vi "数据查询_仪器数据.vi"() -> ()   [LabVIEW 2016, in "数据查询.lvlib"]
uses:
  <vilib>/Utility/miscctls.llb/LVPointTypeDef.ctl
  <vilib>/Utility/miscctls.llb/LVRowAndColumnUnsignedTypeDef.ctl
  <userlib>/_OpenG.lib/array/array.llb/Sort 2D Array (String)__ogtk.vi
panel:
  in  "是否剔除异常数据":bool
  in  "数据类型":string(combo)="全部数据"
  in  "列表框":i32(listbox)
  out "布尔":bool
  in  "页":i32 format="第%.0f页"
  in  "每页条数":i32=1000
  in  "向后按钮":bool
  in  "向前按钮":bool
  in  "导出":bool
  in  "测量模式":string(combo)="全部数据"
  in  "查询":bool
  in  "结束日期":string="2050/01/01"
  in  "起始日期":string="2010/01/01"
  out "数据表":string[][](table)
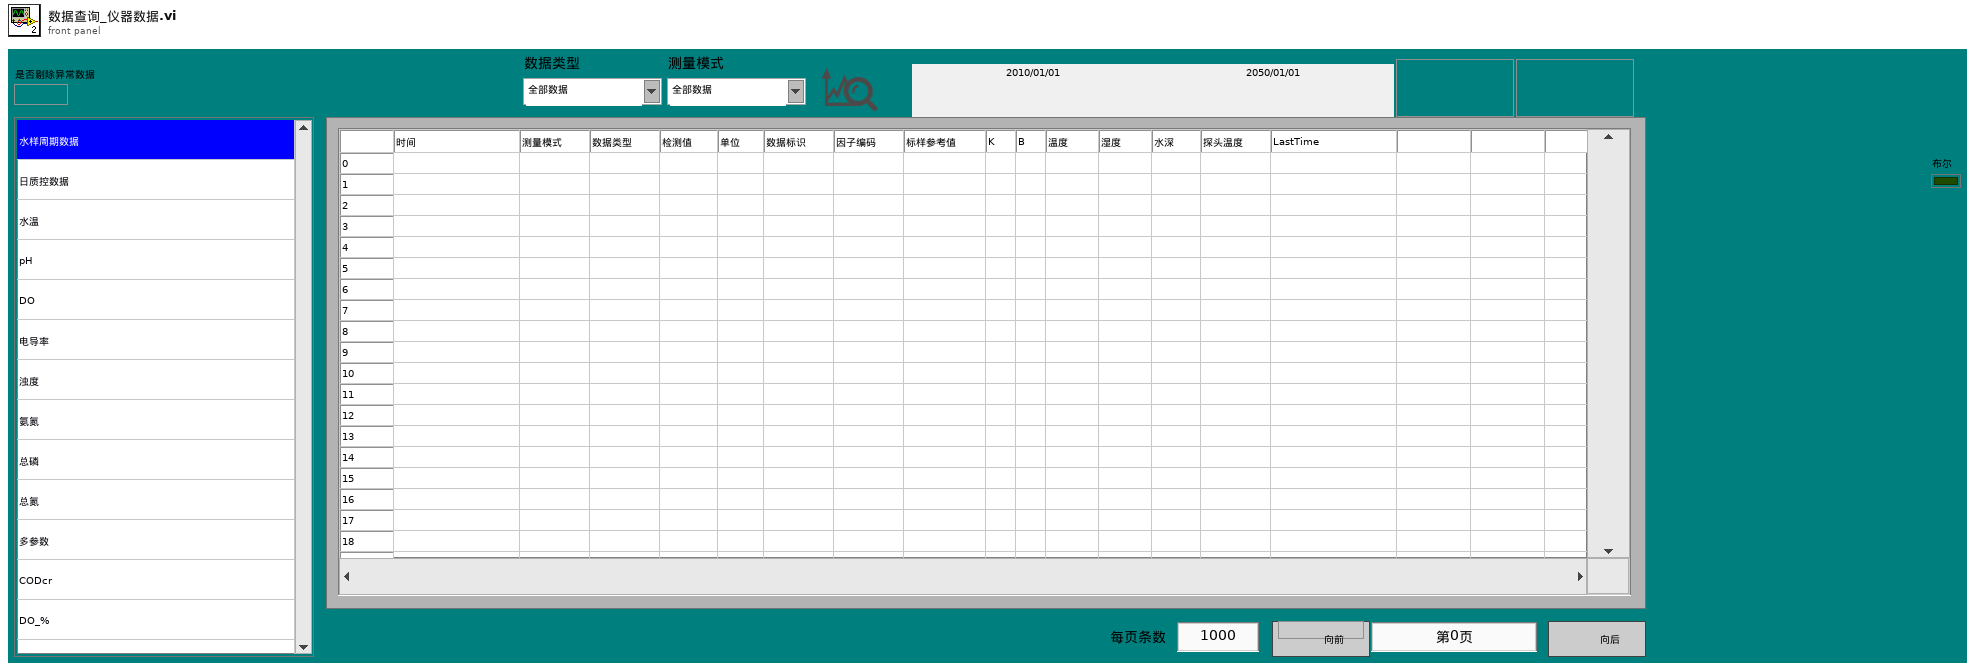
[diagram p1: front panel]
types:
  T1 = typedef "LVPointTypeDef.ctl" = cluster{"Horizontal":i16, "Vertical":i16}
  T2 = typedef "LVDateTimeRec.ctl" = cluster{"秒数的小数部分":dbl, "秒":i32, "分":i32, "时":i32, "日":i32, "月":i32, "年":i32, "天数（周）":i32, "天数（年）":i32, "DST":i32}
  T3 = enum8{"Enabled", "Disabled", "Disabled and Grayed Out"}
  T4 = typedef "LVRowAndColumnUnsignedTypeDef.ctl" = cluster{"Row":u32, "Column":u32}
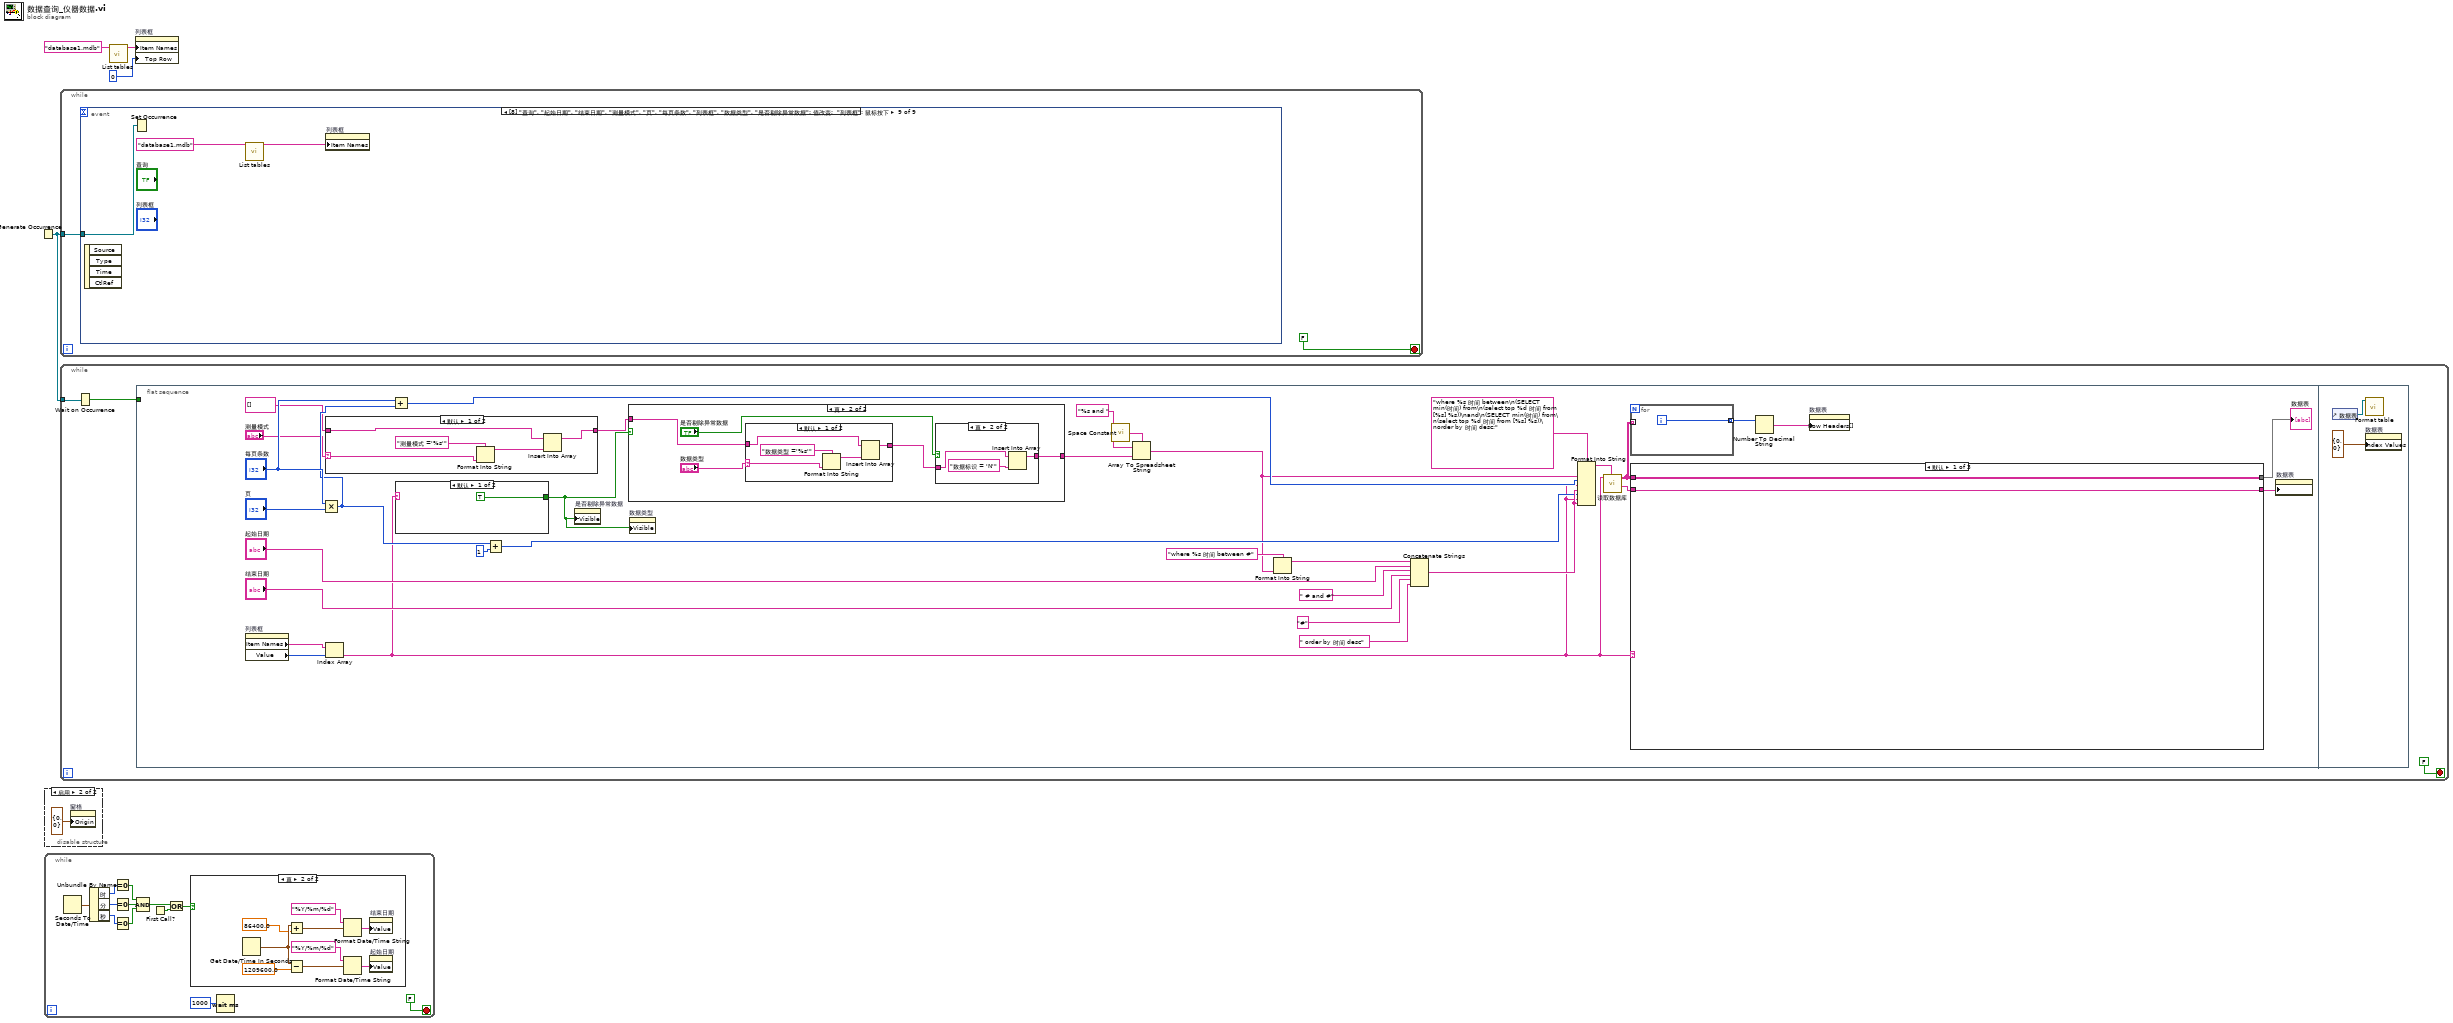
[diagram p0: block diagram]
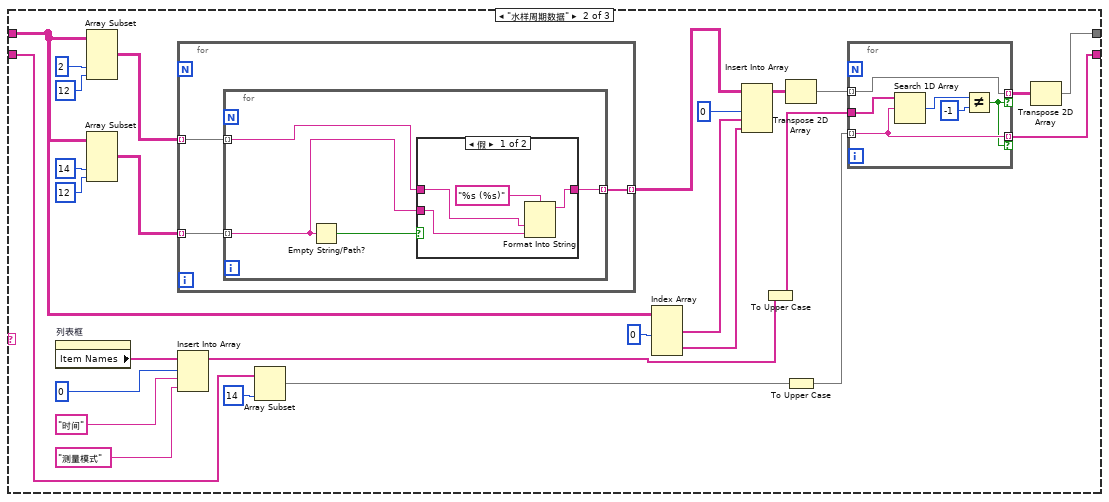
[diagram p7: hidden frame]
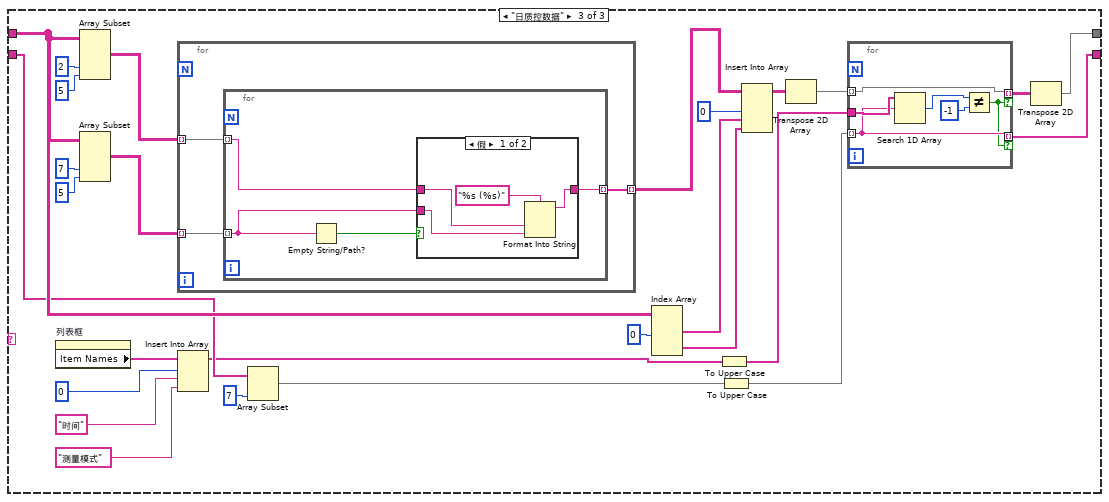
[diagram p9: hidden frame]
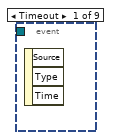
[diagram p12: hidden frame]
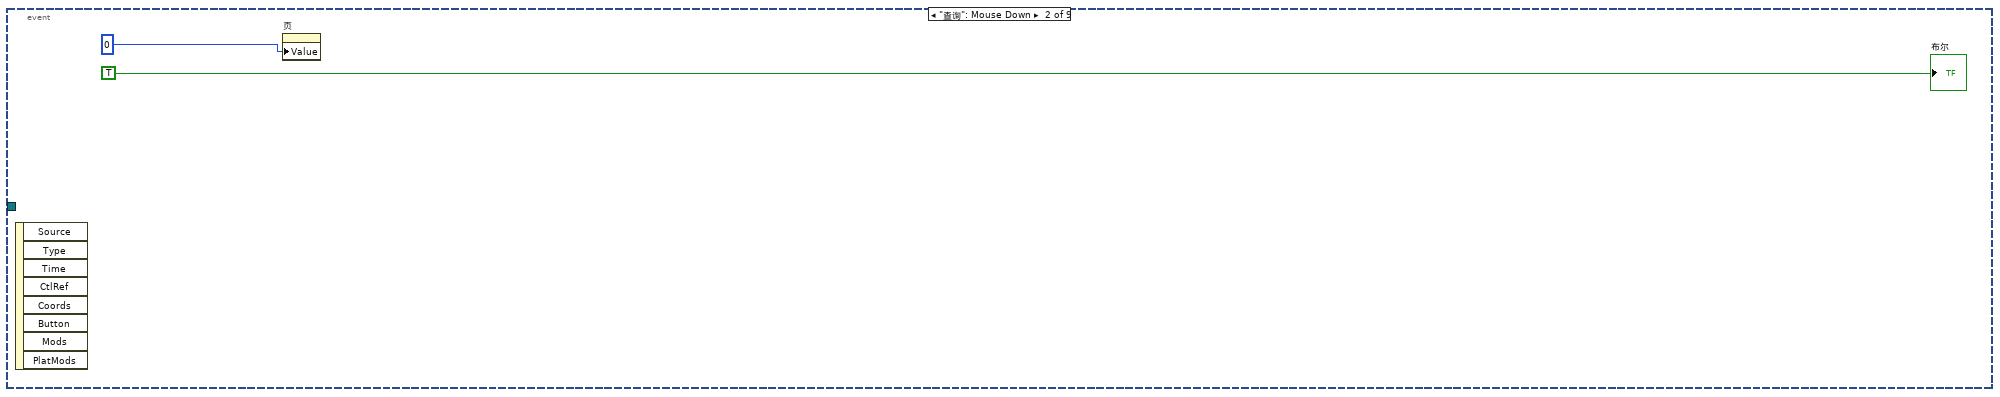
[diagram p13: hidden frame]
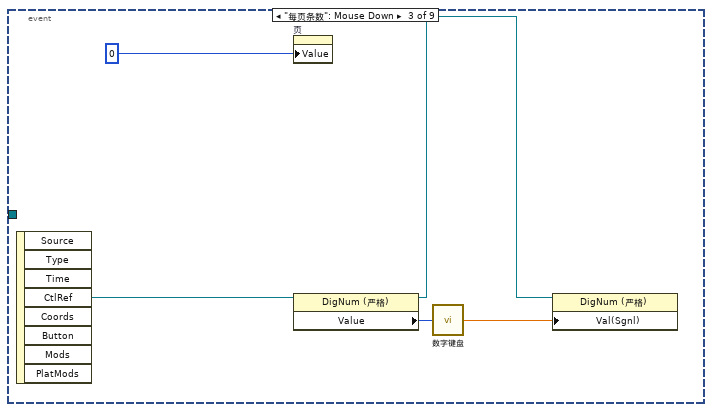
[diagram p14: hidden frame]
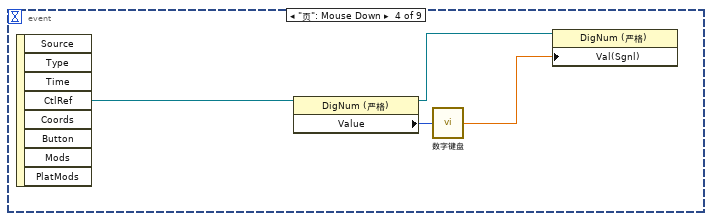
[diagram p15: hidden frame]
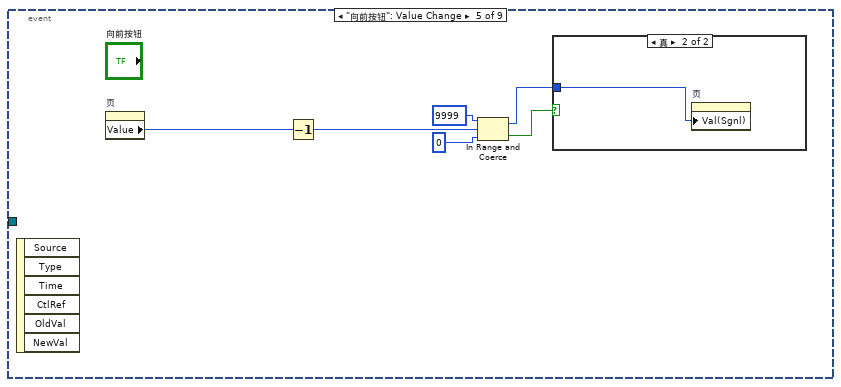
[diagram p16: hidden frame]
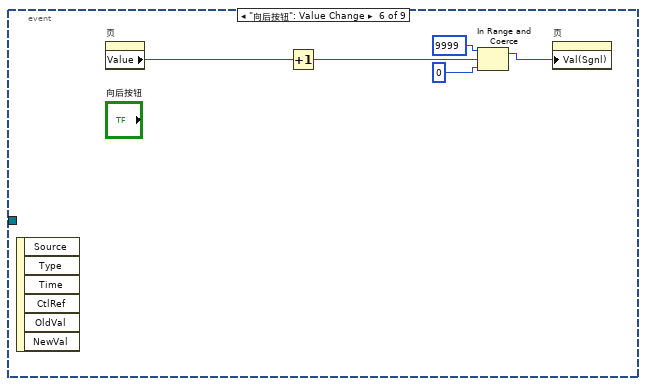
[diagram p18: hidden frame]
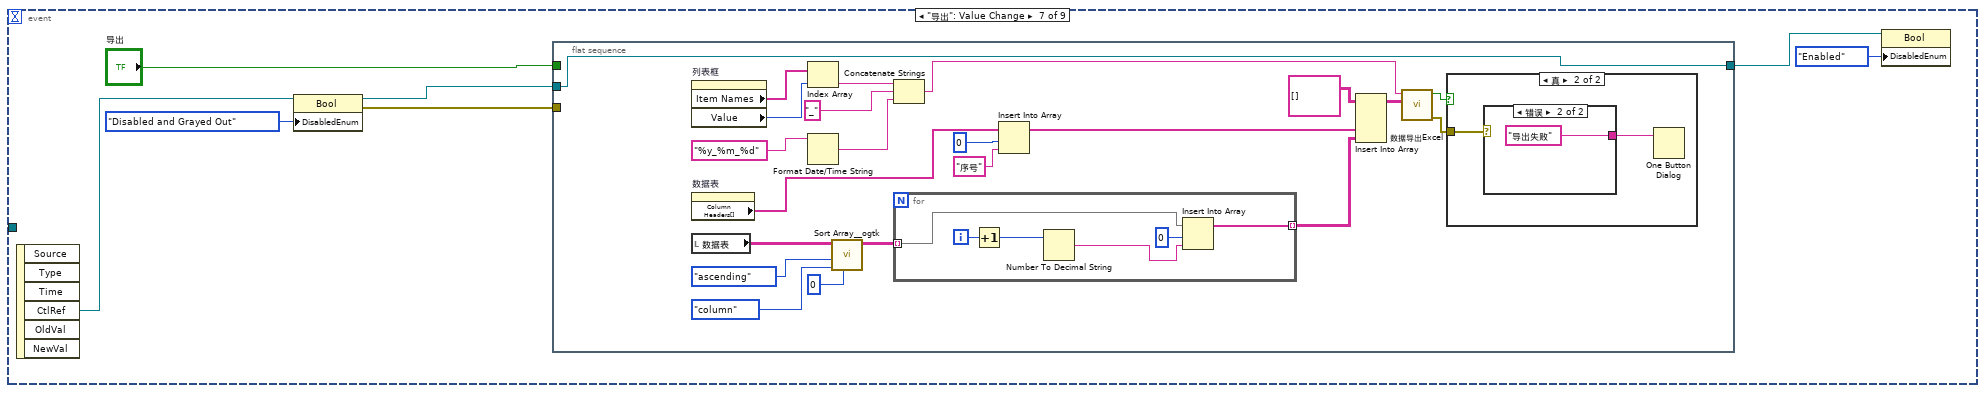
[diagram p19: hidden frame]
diagram:
  n1 = Generate Occurrence() -> (w3:refnum<k4>)
  n2 = disable-structure shown="启用" {
    frame Disabled {
    }
    frame Enabled {
      n3 = property on="窗格" class="Pane"("Origin"=T1 {"Horizontal"=0, "Vertical"=0} ("原点")) -> ()  [unwired: 2 in, 2 out]
    }
  }
  n4 = while {
    stop <- FALSE stop-if-true
    n5 = Seconds To Date/Time() -> (date time rec=w17:T2)  [unwired: 2 in]
    n6 = Unbundle By Name(w17) -> ("时"=w16:i32, "分"=w15:i32, "秒"=w14:i32)
    n7 = Equal To 0?(x=w16) -> (x = 0?=w13:bool)
    n8 = Equal To 0?(x=w15) -> (x = 0?=w12:bool)
    n9 = Equal To 0?(x=w14) -> (x = 0?=w11:bool)
    n10 = Compound Arithmetic op=AND ("复合运算")(w13, w12, w11) -> (w8:bool)
    n11 = First Call?() -> (First Call?: T/F=w7:bool)
    n12 = Or(x=w8, y=w7) -> (x .or. y?=w6:bool)
    n13 = case shown="真" w6 {
      frame False {
      }
      frame True {
        n14 = Get Date/Time In Seconds() -> (seconds since 1Jan1904=w22:timestamp)
        n15 = Add(x=w22, y=86400.0) -> (x+y=w20:timestamp)
        n16 = Subtract(x=w22, y=1209600.0) -> (x-y=w23:timestamp)
        n17 = Format Date/Time String(time format string (%c)="%Y/%m/%d" ("时间格式字符串(%c)"), seconds (now)=w20) -> (date/time string=w19:string)  [unwired: 1 in]
        n18 = Format Date/Time String(time format string (%c)="%Y/%m/%d" ("时间格式字符串(%c)"), seconds (now)=w23) -> (date/time string=w25:string)  [unwired: 1 in]
        n19 = property on="结束日期" class="Str"("Value"=w19) -> ()  [unwired: 2 in, 2 out]
        n20 = property on="起始日期" class="Str"("Value"=w25) -> ()  [unwired: 2 in, 2 out]
      }
    }
    n21 = Wait (ms)(milliseconds to wait=u32 1000 ("等待时间（毫秒）")) -> ()  [unwired: 1 out]
  }
  n22 = while {
    tunnel: w3 -> [w27]
    stop <- FALSE stop-if-true
    n23 = event shown="[8] \"查询\", \"起始日期\", \"结束日期\", \"测量模式\", \"页\", \"每页条数\", \"列表框\", \"数据类型\", \"是否剔除异常数据\": 值改变;  \"列表框\": 鼠标按下" {
      selector: _ -> [_ _ _ _ _ _ _ _ _]
      dyn-events: _ -> [_ _ _ _ _ _ _ _ _]
      timeout: _ -> [_ _ _ _ _ _ _ _ _]
      tunnel: w27 -> [_ _ _ _ _ _ _ _ w96]
      event Timeout {
        n24 = event-data() -> ()  [unwired: 1 in, 3 out]
      }
      event "查询": Mouse Down {
        n25 = event-data() -> ()  [unwired: 1 in, 8 out]
        n26 = property on="页" class="DigNum (严格)"("Value"=0 ("页")) -> ()  [unwired: 2 in, 2 out]
        "布尔" <- TRUE ("布尔")
      }
      event "每页条数": Mouse Down {
        n27 = event-data() -> ("CtlRef"=w32:refnum<vi>)  [unwired: 1 in, 7 out]
        n28 = property on="页" class="DigNum (严格)"("Value"=0 ("页")) -> ()  [unwired: 2 in, 2 out]
        n29 = property class="DigNum (严格)"(reference=w32) -> (reference out=w33:refnum<vi>, "Value"=w35:i32)  [unwired: 1 in, 1 out]
        n30 = call "数字键盘.vi"("OldNumber"=w35) -> ("NewNumber"=w34:sgl)
        n31 = property class="DigNum (严格)"(reference=w33, "Val(Sgnl)"=w34) -> ()  [unwired: 1 in, 2 out]
      }
      event "页": Mouse Down {
        n32 = event-data() -> ("CtlRef"=w36:refnum<vi>)  [unwired: 1 in, 7 out]
        n33 = property class="DigNum (严格)"(reference=w36) -> (reference out=w37:refnum<vi>, "Value"=w39:i32)  [unwired: 1 in, 1 out]
        n34 = call "数字键盘.vi"("OldNumber"=w39) -> ("NewNumber"=w38:sgl)
        n35 = property class="DigNum (严格)"(reference=w37, "Val(Sgnl)"=w38) -> ()  [unwired: 1 in, 2 out]
      }
      event "向前按钮": Value Change {
        n36 = event-data() -> ()  [unwired: 1 in, 6 out]
        n37 = property on="页" class="DigNum (严格)"() -> ("Value"=w45:i32)  [unwired: 2 in, 2 out]
        n38 = Decrement(x=w45) -> (x-1=w44:i32)
        n39 = In Range and Coerce(upper limit=9999 ("上限"), x=w44, lower limit=0 ("下限")) -> (coerced(x)=w41:i32, In Range?=w40:bool)
        n40 = case shown="真" w40 {
          tunnel: w41 -> [_ w46]
          frame False {
          }
          frame True {
            n41 = property on="页" class="DigNum (严格)"("Val(Sgnl)"=w46) -> ()  [unwired: 2 in, 2 out]
          }
        }
      }
      event "向后按钮": Value Change {
        n42 = event-data() -> ()  [unwired: 1 in, 6 out]
        n43 = property on="页" class="DigNum (严格)"() -> ("Value"=w51:i32)  [unwired: 2 in, 2 out]
        n44 = Increment(x=w51) -> (x+1=w50:i32)
        n45 = In Range and Coerce(upper limit=u32 9999 ("上限"), x=w50, lower limit=u32 0 ("下限")) -> (coerced(x)=w47:u32)  [unwired: 1 out]
        n46 = property on="页" class="DigNum (严格)"("Val(Sgnl)"=w47) -> ()  [unwired: 2 in, 2 out]
      }
      event "导出": Value Change {
        n47 = event-data() -> ("CtlRef"=w52:refnum<vi>)  [unwired: 1 in, 5 out]
        n48 = property class="Bool"(reference=w52, "DisabledEnum"=T3."Disabled and Grayed Out" ("禁用")) -> (reference out=w56:refnum<vi>, error out=w57:errorcluster)  [unwired: 1 in]
        n49 = flat-sequence {
          tunnel: w57 -> [_]
          tunnel: [w76] -> w55
          tunnel: w56 -> [w76]
          tunnel: "导出" -> [_]
          frame #0 {
            n50 = property on="列表框" class="LstBox (严格)"() -> ("Item Names"=w61:string[], "Value"=w60:i32)  [unwired: 2 in, 2 out]
            n51 = property on="数据表" class="Tbl (严格)"() -> ("Column Headers[]"=w69:string[])  [unwired: 2 in, 2 out]
            n52 = local read "数据表"() -> (w80:string[][])
            n53 = Index Array(array=w61, index=w60) -> (element=w59:string)
            n54 = Format Date/Time String(time format string (%c)="%y_%m_%d" ("时间格式字符串(%c)")) -> (date/time string=w73:string)  [unwired: 2 in]
            n55 = call-poly <userlib>:"Sort Array__ogtk.vi"("Column/Row to Sort By"=u32 0, "Sort By in"=enum16{"row", "column"}."column", "Order"=enum16{"ascending", "descending"}."ascending", "Array in"=w80) -> ("Sorted Array out"=w62:string[][])  [unwired: 4 in, 3 out]
            n56 = Concatenate Strings(w59, "_" ("字符串"), w73) -> (w71:string)
            n57 = for {
              tunnel: w62 -> [w89] mode=indexing
              tunnel: [w88] -> w66 mode=indexing
              i -> [w90]
              n58 = Increment(x=w90) -> (x+1=w86:i32)
              n59 = Number To Decimal String(number=w86) -> (decimal integer string=w85:string)  [unwired: 1 in]
              n60 = Insert Into Array(array=w89, index=0 ("索引"), new element=w85) -> (w88:string[])
            }
            n61 = Insert Into Array(array=w69, index=0 ("索引"), new element="序号" ("新元素/子数组")) -> (w70:string[])
            n62 = Insert Into Array(array=string[][] [], new element #1=w70, new element #2=w66) -> (w65:string[][])  [unwired: 2 in]
            n63 = call "数据导出Excel.vi"("text data"=w65, "default name"=w71) -> ("error out"=w64:errorcluster, "布尔"=w63:bool)  [unwired: 8 in]
            n64 = case shown="真" w63 {
              tunnel: w64 -> [_ w82]
              frame False {
              }
              frame True {
                n65 = case shown="错误" w82 {
                  tunnel: ["导出成功" ("消息") "导出失败" ("消息")] -> w81
                  frame No Error {
                  }
                  frame Error {
                  }
                }
                n66 = One Button Dialog(message=w81) -> ()  [unwired: 1 in, 1 out]
              }
            }
          }
        }
        n67 = property class="Bool"(reference=w55, "DisabledEnum"=T3."Enabled" ("禁用")) -> ()  [unwired: 1 in, 2 out]
      }
      event "起始日期", "结束日期": Mouse Down {
        n68 = event-data() -> ("CtlRef"=w94:refnum<vi>)  [unwired: 1 in, 7 out]
        n69 = property class="Str"(reference=w94) -> (reference out=w92:refnum<vi>, "Value"=w93:string)  [unwired: 1 in, 1 out]
        n70 = call "日期键盘.vi"("原值"=w93) -> ("x+y"=w91:string)  [unwired: 10 in]
        n71 = property class="Str"(reference=w92, "Val(Sgnl)"=w91) -> ()  [unwired: 1 in, 2 out]
      }
      event "查询", "起始日期", "结束日期", "测量模式", "页", "每页条数", "列表框", "数据类型", "是否剔除异常数据": Value Change; "列表框": Mouse Down {
        n72 = event-data() -> ()  [unwired: 1 in, 4 out]
        n73 = Set Occurrence(w96) -> ()
        n74 = call "List tables.vi"("database"="database1.mdb") -> ("tables"=w95:string[])  [unwired: 9 in, 1 out]
        n75 = property on="列表框" class="LstBox (严格)"("Item Names"=w95) -> ()  [unwired: 2 in, 2 out]
      }
    }
  }
  n76 = while {
    tunnel: w3 -> [w99]
    stop <- FALSE stop-if-true
    n77 = Wait on Occurrence(2:w99) -> (0:w98:bool)  [unwired: 2 in]
    n78 = flat-sequence {
      tunnel: w98 -> [_]
      frame #0 {
        n79 = property on="列表框" class="LstBox (严格)"() -> ("Item Names"=w120:string[], "Value"=w121:i32)  [unwired: 2 in, 2 out]
        n80 = Multiply(x="每页条数", y="页") -> (x*y=w114:i32)
        n81 = case shown="默认" "测量模式" {
          selector: "测量模式" -> [w137 _]
          tunnel: string[] [] -> [w136 w139]
          tunnel: [w134 w139] -> w106
          frame Default {
            n82 = Format Into String(format string="测量模式 ='%s'" ("condition"), w137) -> (resulting string=w135:string)  [unwired: 2 in, 1 out]
            n83 = Insert Into Array(array=w136, new element=w135) -> (w134:string[])  [unwired: 1 in]
          }
          frame "全部数据" {
          }
        }
        n84 = Index Array(array=w120, index=w121) -> (element=w109:string)
        n85 = Add(x="每页条数", y=w114) -> (x+y=w112:i32)
        n86 = case shown="默认" w109 {
          tunnel: [TRUE _] -> w101
          frame Default {
          }
          frame "MPPT12", "MPPT24", "电压", "多参数", "环境参数", "集成干预测试", "加标回收率", "日质控数据", "湿度", "室温", "水样周期数据", "移位距离" {
          }
        }
        n87 = Add(x=w114, y=u32 1) -> (x+y=w111:u32)
        n88 = property on="是否剔除异常数据" class="Bool (严格)"("Visible"=w101) -> ()  [unwired: 2 in, 2 out]
        n89 = case shown="真" w101 {
          tunnel: [w140 w141] -> w103
          tunnel: w106 -> [w140 w142]
          frame False {
          }
          frame True {
            n90 = case shown="默认" "数据类型" {
              selector: "数据类型" -> [w149 _]
              tunnel: w142 -> [w148 w151]
              tunnel: [w146 w151] -> w143
              frame Default {
                n91 = Format Into String(format string="数据类型 ='%s'" ("condition"), w149) -> (resulting string=w147:string)  [unwired: 2 in, 1 out]
                n92 = Insert Into Array(array=w148, new element=w147) -> (w146:string[])  [unwired: 1 in]
              }
              frame "全部数据" {
              }
            }
            n93 = case shown="真" "是否剔除异常数据" {
              tunnel: w143 -> [w152 w155]
              tunnel: [w152 w153] -> w141
              frame False {
              }
              frame True {
                n94 = Insert Into Array(array=w155, new element="数据标识 = 'N'" ("condition")) -> (w153:string[])  [unwired: 1 in]
              }
            }
          }
        }
        n95 = property on="数据类型" class="CmbBox"("Visible"=w101) -> ()  [unwired: 2 in, 2 out]
        n96 = call <vilib>:"Space Constant.vi"() -> ("String"=w105:string)
        n97 = Array To Spreadsheet String(delimiter (Tab)=w105, array=w103, 3:"%s and " ("格式字符串")) -> (spreadsheet string=w102:string)
        n98 = Format Into String(format string="where %s 时间 between #" ("condition"), w102) -> (resulting string=w127:string)  [unwired: 2 in, 1 out]
        n99 = Concatenate Strings(w127, "起始日期", " # and #" ("condition"), "结束日期", "#" ("condition"), " order by 时间 desc" ("字符串")) -> (w125:string)
        n100 = Format Into String(format string="where %s 时间 between\n(SELECT min(时间) from\n(select top %d 时间 from [%s] %s))\nand\n(SELECT min(时间) from\n(select top %d 时间 from [%s] %s))\norder by 时间 desc;" ("格式字符串"), w102, w112, w109, w125, w111, w109, w125) -> (resulting string=w124:string)  [unwired: 2 in, 1 out]
        n101 = call "读取数据库.vi"("condition"=w124, "组合框"=w109) -> ("columns"=w118:string[], "表格"=w117:string[][])  [unwired: 6 in, 2 out]
        n102 = for {
          tunnel: w117 -> [_] mode=indexing
          tunnel: [w249] -> w129 mode=indexing
          i -> [w249]
        }
        n103 = case shown="默认" w109 {
          tunnel: [w158 w163 w208] -> w119
          tunnel: w118 -> [w157 w174 w219]
          tunnel: w117 -> [w158 w175 w220]
          tunnel: [w157 w171 w216] -> w116
          frame Default {
          }
          frame "水样周期数据" {
            n104 = property on="列表框" class="LstBox (严格)"() -> ("Item Names"=w167:string[])  [unwired: 2 in, 2 out]
            n105 = Array Subset(array=w175, index (col)=2 ("索引"), length (col)=12 ("长度")) -> (w176:string[][])  [unwired: 2 in]
            n106 = Array Subset(array=w175, index (col)=14 ("长度"), length (col)=12 ("长度")) -> (w179:string[][])  [unwired: 2 in]
            n107 = for {
              tunnel: [w194] -> w185 mode=indexing
              tunnel: w176 -> [w193] mode=indexing
              tunnel: w179 -> [w192] mode=indexing
              n108 = for {
                tunnel: w193 -> [w197] mode=indexing
                tunnel: [w198] -> w194 mode=indexing
                tunnel: w192 -> [w196] mode=indexing
                n109 = Empty String/Path?(string/path=w196) -> (empty?=w195:bool)
                n110 = case shown="假" w195 {
                  tunnel: w197 -> [w202 w203]
                  tunnel: w196 -> [w201 _]
                  tunnel: [w199 w203] -> w198
                  frame False {
                    n111 = Format Into String(format string="%s (%s)" ("格式字符串"), w202, w201) -> (resulting string=w199:string)  [unwired: 2 in, 1 out]
                  }
                  frame True {
                  }
                }
              }
            }
            n112 = Insert Into Array(array=w167, index=0 ("索引"), new element #1="时间" ("新元素/子数组"), new element #2="测量模式" ("新元素/子数组")) -> (w168:string[])
            n113 = Array Subset(array=w174, length=14 ("长度")) -> (w172:string[])  [unwired: 1 in]
            n114 = Index Array(array=w175, index (col) #1=0 ("禁用的索引 (列)")) -> (element #1=w173:string[], element #2=w161:string[])  [unwired: 3 in]
            n115 = Insert Into Array(array=w185, index (col)=0 ("禁用的索引 (列)"), new element #1=w173, new element #2=w161) -> (w170:string[][])  [unwired: 1 in]
            n116 = To Upper Case(1:w168) -> (0:w160:string[])
            n117 = Transpose 2D Array(2D array=w170) -> (transposed array=w169:string[][])
            n118 = To Upper Case(1:w172) -> (0:w159:string[])
            n119 = for {
              tunnel: w159 -> [w190] mode=indexing
              tunnel: w169 -> [w186] mode=indexing
              tunnel: w160 -> [w191]
              tunnel: [w190] -> w171 mode=indexing if=w187
              tunnel: [w186] -> w164 mode=indexing if=w187
              n120 = Search 1D Array(1D array=w191, element=w190) -> (index of element=w188:i32)  [unwired: 1 in]
              n121 = Not Equal?(x=w188, y=-1) -> (x != y?=w187:bool)
            }
            n122 = Transpose 2D Array(2D array=w164) -> (transposed array=w163:string[][])
          }
          frame "日质控数据" {
            n123 = property on="列表框" class="LstBox (严格)"() -> ("Item Names"=w212:string[])  [unwired: 2 in, 2 out]
            n124 = Array Subset(array=w220, index (col)=2 ("索引"), length (col)=5 ("长度")) -> (w221:string[][])  [unwired: 2 in]
            n125 = Array Subset(array=w220, index (col)=7 ("长度"), length (col)=5 ("长度")) -> (w224:string[][])  [unwired: 2 in]
            n126 = for {
              tunnel: [w239] -> w230 mode=indexing
              tunnel: w221 -> [w238] mode=indexing
              tunnel: w224 -> [w237] mode=indexing
              n127 = for {
                tunnel: w238 -> [w242] mode=indexing
                tunnel: [w243] -> w239 mode=indexing
                tunnel: w237 -> [w241] mode=indexing
                n128 = Empty String/Path?(string/path=w241) -> (empty?=w240:bool)
                n129 = case shown="假" w240 {
                  tunnel: w242 -> [w247 w248]
                  tunnel: w241 -> [w246 _]
                  tunnel: [w244 w248] -> w243
                  frame False {
                    n130 = Format Into String(format string="%s (%s)" ("格式字符串"), w247, w246) -> (resulting string=w244:string)  [unwired: 2 in, 1 out]
                  }
                  frame True {
                  }
                }
              }
            }
            n131 = Insert Into Array(array=w212, index=0 ("索引"), new element #1="时间" ("新元素/子数组"), new element #2="测量模式" ("新元素/子数组")) -> (w213:string[])
            n132 = Array Subset(array=w219, length=7 ("长度")) -> (w217:string[])  [unwired: 1 in]
            n133 = Index Array(array=w220, index (col) #1=0 ("禁用的索引 (列)")) -> (element #1=w218:string[], element #2=w206:string[])  [unwired: 3 in]
            n134 = To Upper Case(1:w213) -> (0:w205:string[])
            n135 = To Upper Case(1:w217) -> (0:w204:string[])
            n136 = Insert Into Array(array=w230, index (col)=0 ("禁用的索引 (列)"), new element #1=w218, new element #2=w206) -> (w215:string[][])  [unwired: 1 in]
            n137 = Transpose 2D Array(2D array=w215) -> (transposed array=w214:string[][])
            n138 = for {
              tunnel: w204 -> [w235] mode=indexing
              tunnel: w214 -> [w231] mode=indexing
              tunnel: w205 -> [w236]
              tunnel: [w235] -> w216 mode=indexing if=w232
              tunnel: [w231] -> w209 mode=indexing if=w232
              n139 = Search 1D Array(1D array=w236, element=w235) -> (index of element=w233:i32)  [unwired: 1 in]
              n140 = Not Equal?(x=w233, y=-1) -> (x != y?=w232:bool)
            }
            n141 = Transpose 2D Array(2D array=w209) -> (transposed array=w208:string[][])
          }
        }
        "数据表" <- w119
        n142 = Number To Decimal String(number=w129) -> (decimal integer string=w128:string[])  [unwired: 1 in]
        n143 = property on="数据表" class="Tbl (严格)"("Row Headers[]"=w128) -> ()  [unwired: 2 in, 2 out]
        n144 = property on="数据表" class="Tbl (严格)"("Column Headers[]"=w116) -> ()  [unwired: 2 in, 2 out]
      }
      frame #1 {
        n145 = control-ref of="数据表"() -> (w250:refnum<vi>)
        n146 = call "Format table.vi"("Table输入"=w250) -> ()  [unwired: 11 in]
        n147 = property on="数据表" class="Tbl (严格)"("Index Values"=T4 {"Row"=0, "Column"=0} ("索引值")) -> ()  [unwired: 2 in, 2 out]
      }
    }
  }
  n148 = call "List tables.vi"("database"="database1.mdb") -> ("tables"=w2:string[])  [unwired: 9 in, 1 out]
  n149 = property on="列表框" class="LstBox (严格)"("Item Names"=w2, "Top Row"=0 ("顶行")) -> ()  [unwired: 2 in, 2 out]
